vi "Engine - Generic - Port Injector Host.vi"() -> ()   [LabVIEW 2015, in "ECS-Host.lvlib"]
uses:
  ECS-Host.lvlib
  <vilib>/addons/Software Calibration Management/XControls/TBL1D.xctl
panel:
  out "Timing_Des":sgl[](array[numeric]) caption="[DBTDC]"
  in  "AutoTiming_E":bool caption="AutoTiming"
  in  "IVC":sgl caption="[]"
  in  "CamSwitch":bool
  in  "IVO":sgl caption="[]"
  in  "PsnMode":u8
  in  "_Position Mode":bool[](array[boolean]) caption="Position Mode"
  in  "PulseWidth_Max":sgl caption="[]"
  in  "PulseWidth_Man":sgl[](array[numeric]) caption="[msec]"
  out "InjQty":sgl[](array[numeric]) caption="[mg/cyc]"
  in  "MAPCorrFactor_E":bool caption="Enable Inj"
  in  "MAPCorrFactor_Tbl":cluster{"X":sgl[], "Y":sgl[]}(xcontrol)
  in  "InjectorOpenTime_Tbl":cluster{"X":sgl[], "Y":sgl[]}(xcontrol)
  in  "PFIFuelDensity":sgl caption="[]"
  in  "PFIInjectorFlowRate":sgl caption="[]"
  in  "InjectorOpenTime_Gain":sgl caption="[]"
  out "InjectorOpenTime_TblOut":sgl caption="[]"
  in  "PulseWidth_ManE":bool caption="Man Enable"
  out "_FuelPulseWidth Cyl Index":string[](array[string]) caption="[]"
  out "PulseWidth_Des":sgl[](array[numeric]) caption="[msec]"
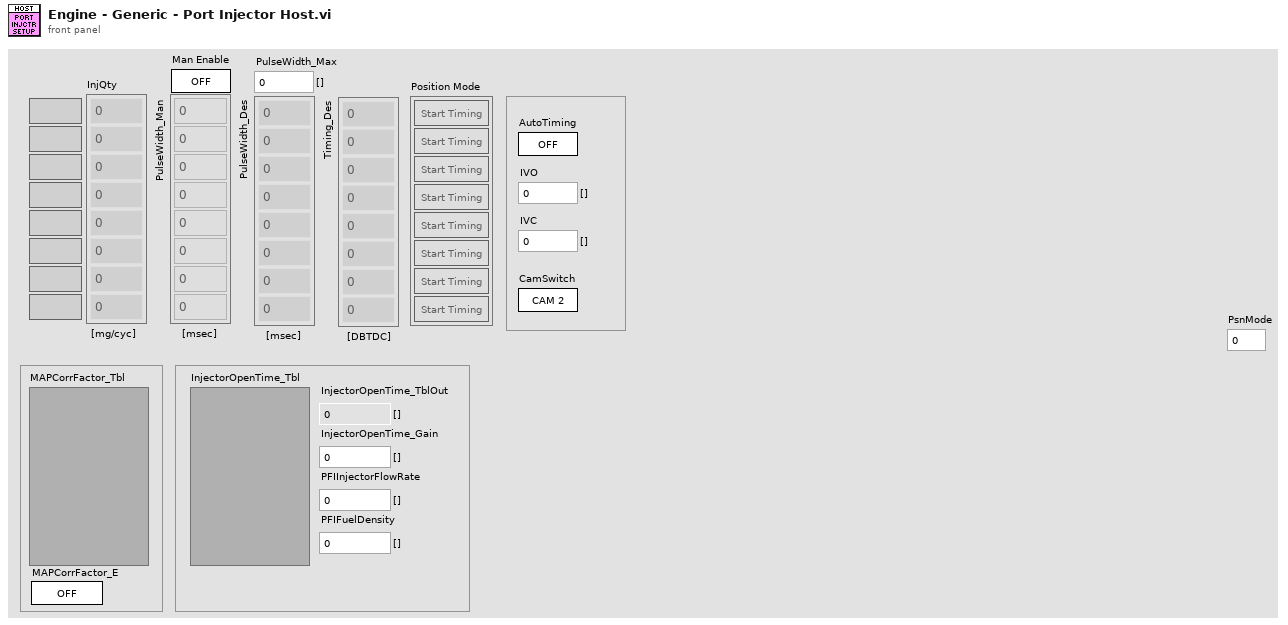
[diagram p1: front panel]
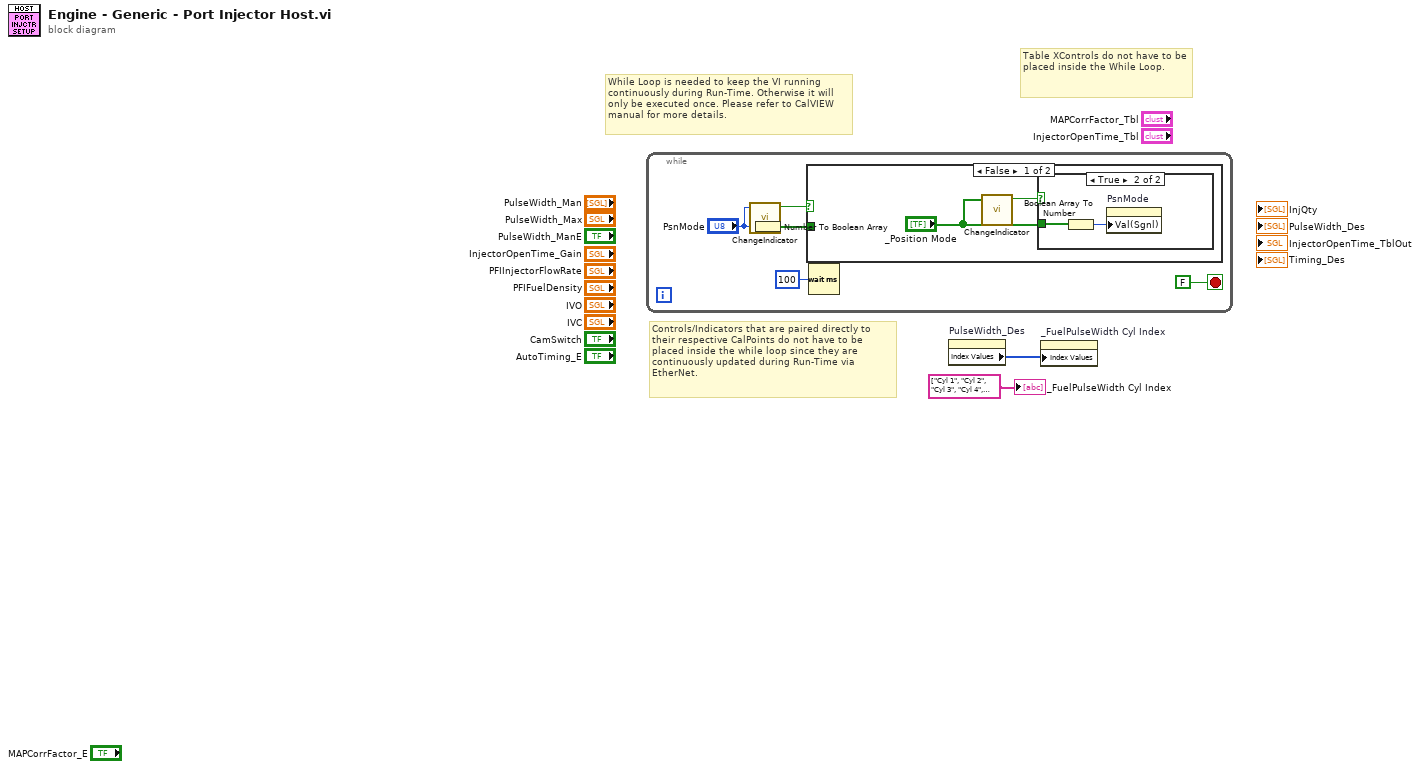
[diagram p0: block diagram]
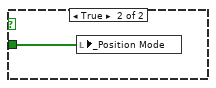
[diagram p3: hidden frame]
diagram:
  # "Controls/Indicators that are paired directly to their respective CalPoints do not have to be placed inside the while loop since they are continuously updated during Run-Time via EtherNet."
  # "Table XControls do not have to be placed inside the While Loop."
  # "While Loop is needed to keep the VI running\ncontinuously during Run-Time. Otherwise it will only be executed once. Please refer to CalVIEW manual for more details."
  n1 = while {
    stop <- FALSE stop-if-true
    n2 = call "ChangeIndicator.vi"("Input"="PsnMode") -> ("Change"=w4:bool)  [unwired: 9 in]
    n3 = Number To Boolean Array(number="PsnMode") -> (Boolean array=w5:bool[])
    n4 = case shown="False" w4 {
      tunnel: w5 -> [_ w12]
      frame False {
        n5 = call "ChangeIndicator.vi"("Input"="_Position Mode") -> ("Change"=w9:bool)  [unwired: 9 in]
        n6 = case shown="True" w9 {
          tunnel: "_Position Mode" -> [_ w10]
          frame False {
          }
          frame True {
            n7 = Boolean Array To Number(Boolean array=w10) -> (number=w11:u8)
            n8 = property on="PsnMode" class="DigNum (strict)"("Val(Sgnl)"=w11) -> ()  [unwired: 2 in, 2 out]
          }
        }
      }
      frame True {
        n9 = local write "_Position Mode"(w12) -> ()
      }
    }
    n10 = Wait (ms)(milliseconds to wait=u32 100) -> ()  [unwired: 1 out]
  }
  n11 = property on="PulseWidth_Des" class="Arr (strict)"() -> ("Index Values"=w1:u32[])  [unwired: 2 in, 2 out]
  n12 = property on="_FuelPulseWidth Cyl Index" class="Arr (strict)"("Index Values"=w1) -> ()  [unwired: 2 in, 2 out]
  "_FuelPulseWidth Cyl Index" <- string[] ["Cyl 1", "Cyl 2", "Cyl 3", "Cyl 4", "Cyl 5", "Cyl 6", "Cyl 7", "Cyl 8"] ("FuelPulseWidth 3")
